vi "차선 인식(선형 피팅).vi"() -> ()   [LabVIEW 2018]
uses:
  <vilib>/Math Plots/3D Math Plots/3D Scatter/3D Scatter XCtrl/3D Scatter.xctl
  <vilib>/Analysis/Matrix/Datatypes/RealMatrix.ctl
  <vilib>/Analysis/Matrix/Numeric/Conversions/Array To Matrix - RA.vi
  <vilib>/Analysis/Matrix/Numeric/Multiply/Multiply - RM,RM.vi
  <vilib>/Analysis/Matrix/Numeric/Conversions/Matrix To Array - RM.vi
  <vilib>/Math Plots/3D Math Plots/3D Scatter/3D Scatter Datatype/Public/Plot Helper (Vector).vi
  <vilib>/Math Plots/3D Math Plots/3D Scatter/3D Scatter Datatype/3D Scatter Datatype.lvclass
  <vilib>/Analysis/Matrix/NI_Matrix.lvlib
  <vilib>/Analysis/NI_AALPro.lvlib
panel:
  out "노이즈 제거 후 오른쪽 차선":cluster{dbl[], dbl[]}(graph)
  out "노이즈 제거 후 전체 차선":cluster{dbl[], dbl[]}(graph)
  out "노이즈 제거 후 왼쪽 차선":cluster{dbl[], dbl[]}(graph)
  out "왼쪽 차선(중점":cluster{dbl[], dbl[]}(graph)
  out "오른쪽 차선(중점)":cluster{dbl[], dbl[]}(graph)
  out "클러스터링 후 (중점)":cluster{dbl[], dbl[]}(graph)
  out "전체 차선":cluster{dbl[], dbl[]}(graph)
  out "왼쪽 차선":cluster{dbl[], dbl[]}(graph)
  out "오른쪽 차선":cluster{dbl[], dbl[]}(graph)
  out "왼쪽 차선(모든 점)":cluster{dbl[], dbl[]}(graph)
  out "오른쪽 차선(모든 점)":cluster{dbl[], dbl[]}(graph)
  out "반사율 꼬깔콘":cluster{dbl[], dbl[]}(graph)
  out "101이상 반사율":u8[](array[numeric])
  out "95~100반사율 배열":cluster{dbl, dbl, dbl, u8}[](array[cluster])
  out "반사율 xy(차선x)":cluster{dbl[], dbl[]}(graph)
  out "60미만 반사율":u8[](array[numeric])
  out "95이상 반사율":u8[](array[numeric])
  out "반사율 xy":cluster{dbl[], dbl[]}(graph)
  out "XZ 2":cluster{dbl[], dbl[]}(graph)
  out "클러스터링 후(모든 점)":cluster{dbl[], dbl[]}(graph)
  out "배열 5":cluster{dbl, dbl, dbl, i32}[](array[cluster])
  out "배열 2":u8[](array[numeric])
  out "XY 그래프":cluster{dbl[], dbl[]}(graph)
  out "azimuth 배열 사이즈":i32
  out "XZ":cluster{dbl[], dbl[]}(graph)
  out "YZ":cluster{dbl[], dbl[]}(graph)
  out "XY":cluster{dbl[], dbl[]}(graph)
  out "3D Scatter":refnum<class "3D Plot Datatype.lvclass">[](xcontrol)
  out "범위내의 X,Y,Z,반사율":cluster{dbl, dbl, dbl, u8}[](array[cluster])
  out "substring":string
  out "Array":string[](array[string])
  out "distance":dbl[](array[numeric])
  out "output array":u8[](array[numeric])
  in  "Boolean":bool
  out "xz":cluster{dbl[], dbl[]}(graph)
  out "yz":cluster{dbl[], dbl[]}(graph)
  out "XY Graph":cluster{dbl[], dbl[]}(graph)
  out "unsigned byte array":u8[][][](array[numeric])
  out "azimuth":dbl[](array[numeric])
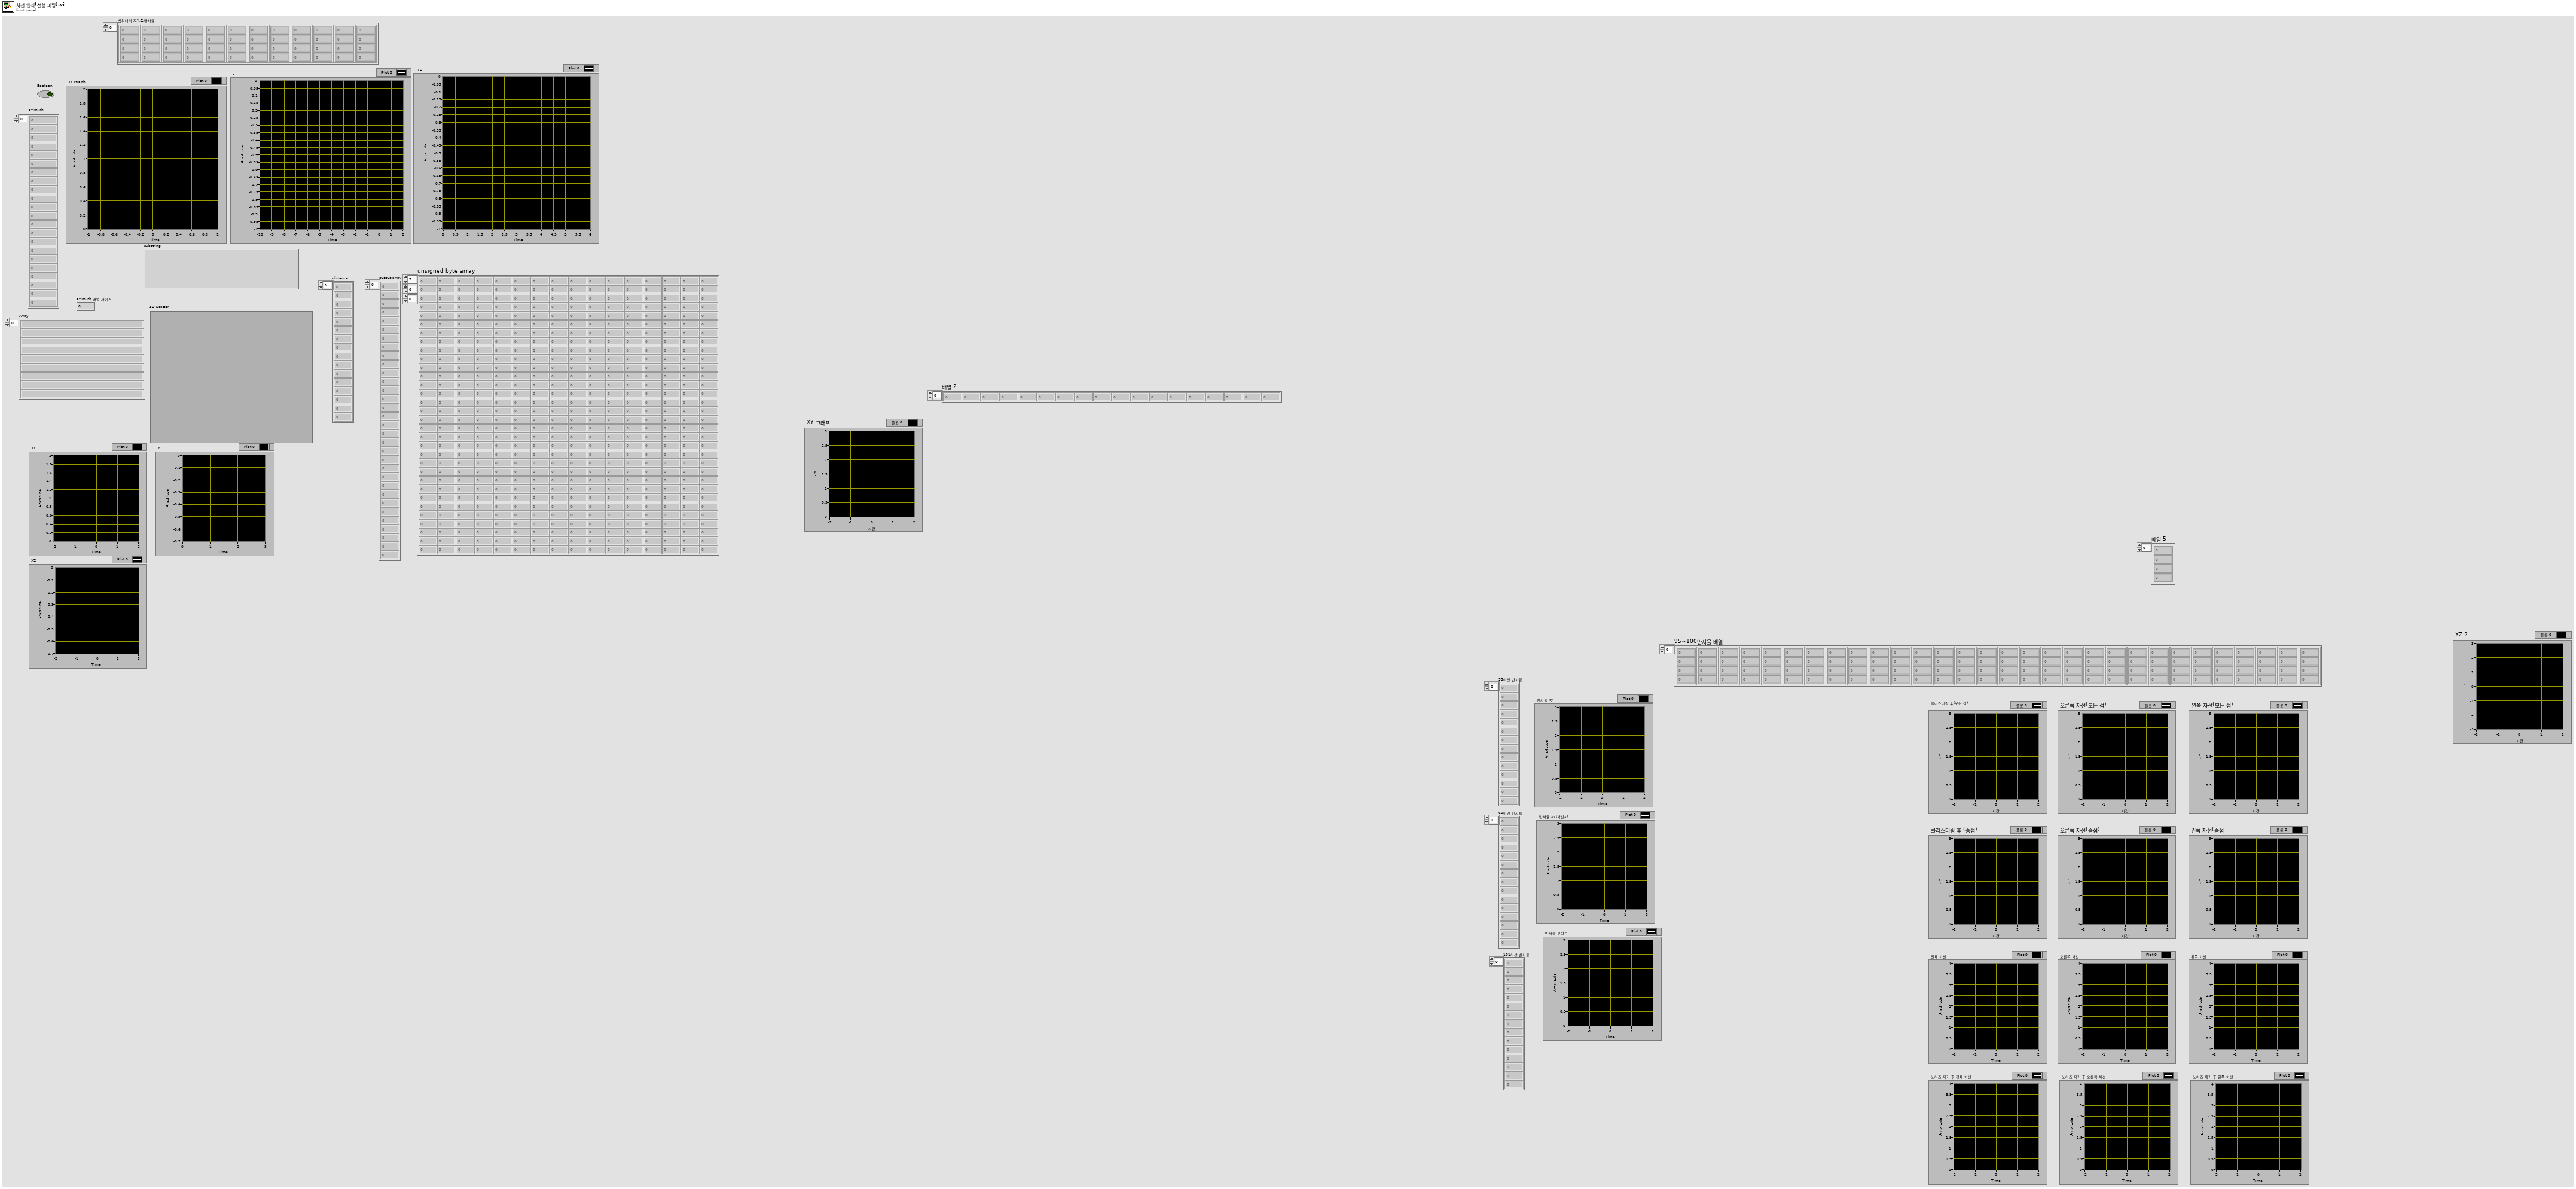
[diagram p1: front panel]
types:
  T1 = typedef "NI_Matrix.lvlib/RealMatrix.ctl" = dbl[][]
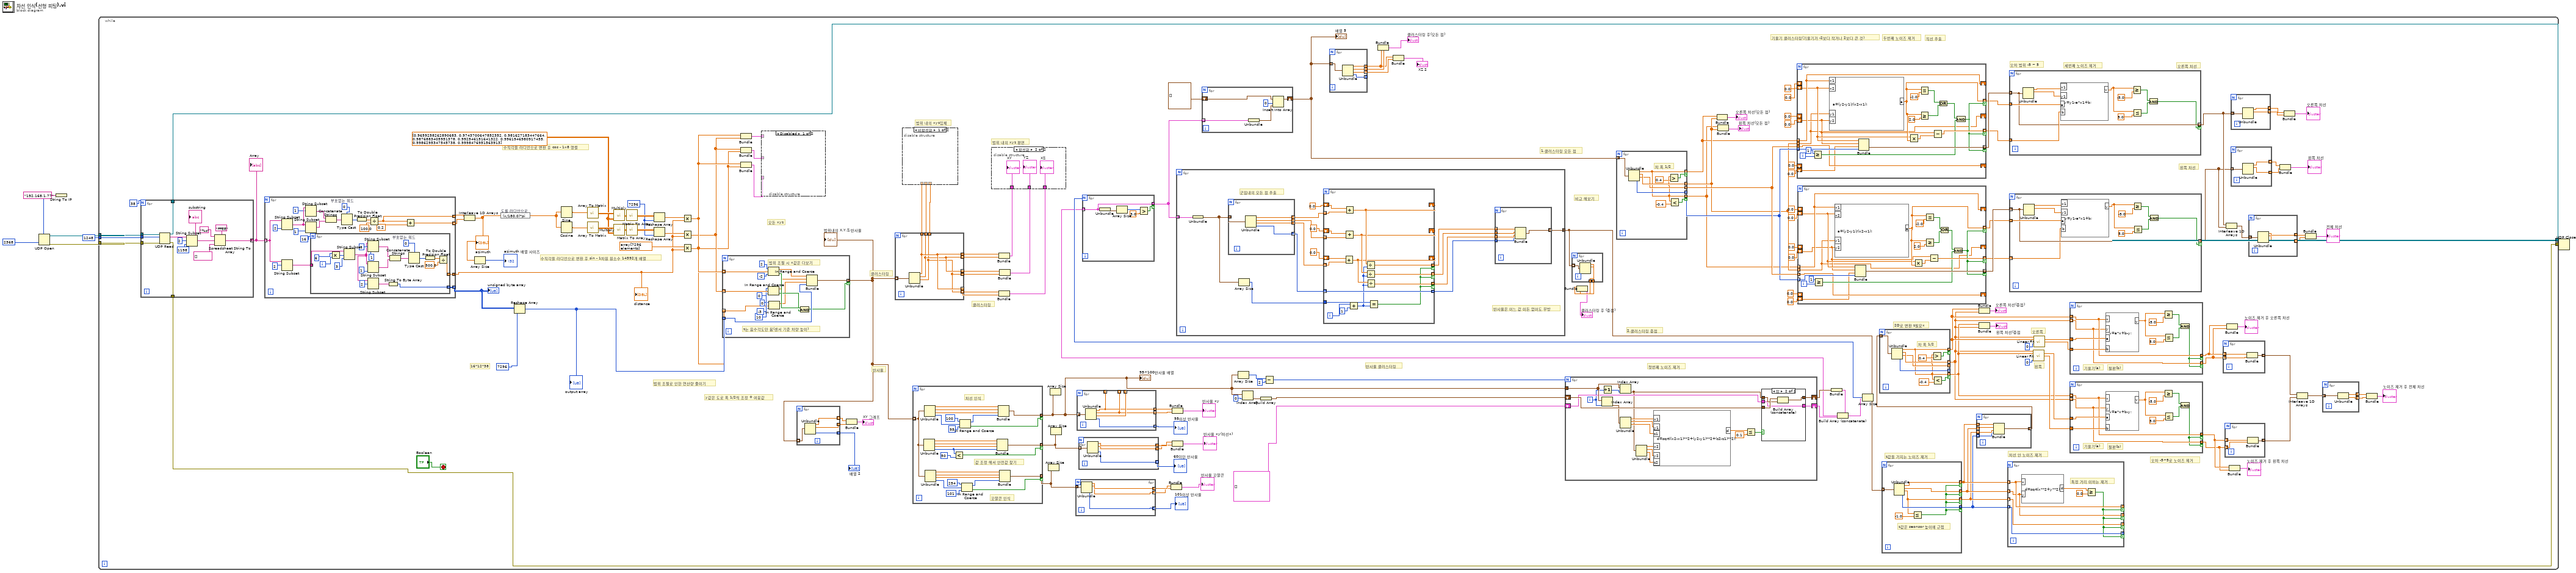
[diagram p0: block diagram]
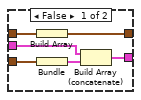
[diagram p2: hidden frame]
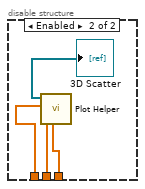
[diagram p4: hidden frame]
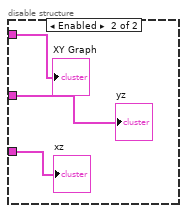
[diagram p5: hidden frame]
diagram:
  n1 = String To IP(1:"192.168.1.77") -> (0:w7:u32)
  n2 = UDP Open(7:w7, 11:2368) -> (port=w5:refnum<k16>, 0:w3:errorcluster)  [unwired: 3 in, 1 out]
  n3 = while {
    tunnel: w5 -> [w164]
    tunnel: 1248 -> [w163]
    tunnel: w3 -> [w162]
    tunnel: [w151] -> w2
    tunnel: [w134] -> w1
    stop <- "Boolean" stop-if-true
    w125 = 7296 ("차원 크기")
    w122 = T1 [[0.9659258262890683, 0.9743700647852352, 0.981627183447664, 0.9876883405951378, 0.992546151641322, 0.9961946980917455, 0.9986295347545738, 0.9998476951563913]] ("전치 행렬")
    # "오차 -5~5로 노이즈 제거"
    # "2D로 변환 z필요x"
    # "왼쪽"
    # "오른쪽"
    # "차선 안 노이즈 제거"
    # "z값을 가지는 노이즈 제거"
    # "2.클러스터링 중점"
    # "1.클러스터링 모든 점"
    # "비교 해보기"
    # "왼쪽 차선"
    # "오른쪽 차선"
    # "오차 범위 -5 ~ 5"
    # "세번째 노이즈 제거"
    # "직선 추출"
    # "기울기 클러스터링(기울기가 -2보다 작거나 2보다 큰 것)"
    # "두번째 노이즈 제거"
    # "첫번째 노이즈 제거"
    # "y값은 도로 폭 1/2씩 조정 + 여윳값"
    # "반사율 클러스터링"
    # "범위 조절로 인한 연산량 줄이기"
    # "반사율"
    # "클러스터링"
    # "수직각을 라디언으로 변환 후 cos - 1x8 행렬"
    # "클러스터링"
    # "범위 내의 xyz 평면"
    # "범위 내의 xyz입체"
    # "모든 xyz"
    # "16*12*38"
    # "수직각을 라디언으로 변환 후 sin - 1차원 원소수 14592개 배열"
    n4 = for {
      N: 38 -> [_]
      tunnel: w164 -> [w518]
      tunnel: w163 -> [w517]
      tunnel: w162 -> [w516]
      tunnel: [w512] -> w151
      tunnel: [w507] -> w161 mode=concatenating
      tunnel: [w506] -> w134
      n5 = UDP Read(connection ID=w518, max size (548)=w517, 8:w516) -> (data out=w515:string, error out=w512:errorcluster, 3:w506:refnum<k16>)  [unwired: 1 in, 2 out]
      n6 = String Subset(string=w515, offset (0)=2, length (rest)=1198) -> (substring=w511:string)
      "substring" <- w511
      n7 = Spreadsheet String To Array(delimiter (Tab)="FFEE", format string="%s", spreadsheet string=w511, array type (2D Dbl)=string[] []) -> (array=w507:string[])
    }
    "Array" <- w161
    n8 = for {
      tunnel: w161 -> [w485] mode=indexing
      tunnel: [w472] -> w159 mode=indexing
      tunnel: [w471] -> w160 mode=indexing
      tunnel: [w468] -> w118 mode=concatenating
      tunnel: [w467] -> w158 mode=indexing
      w466 = u16 0  # 부호없는 워드
      n9 = String Subset(string=w485, offset (0)=2) -> (substring=w469:string)  [unwired: 1 in]
      n10 = String Subset(string=w485, length (rest)=2) -> (substring=w482:string)  [unwired: 1 in]
      n11 = String Subset(string=w482, offset (0)=1) -> (substring=w479:string)  [unwired: 1 in]
      n12 = String Subset(string=w482, length (rest)=1) -> (substring=w478:string)  [unwired: 1 in]
      n13 = for {
        N: 16 -> [_]
        tunnel: w469 -> [w505]
        tunnel: [w492] -> w468 mode=indexing
        tunnel: [w488] -> w467 mode=indexing
        i -> [w504]
        w486 = u16 0  # 부호없는 워드
        n14 = Multiply(x=6, y=w504) -> (x*y=w502:i32)
        n15 = String Subset(string=w505, offset (0)=w502, length (rest)=3) -> (substring=w491:string)
        n16 = String Subset(string=w491, offset (0)=2) -> (substring=w489:string)  [unwired: 1 in]
        n17 = String Subset(string=w491, offset (0)=1, length (rest)=1 ("length (rest)")) -> (substring=w498:string)
        n18 = String Subset(string=w491, length (rest)=1) -> (substring=w497:string)  [unwired: 1 in]
        n19 = String To Byte Array(string=w489) -> (unsigned byte array=w488:u8[])
        n20 = Concatenate Strings(w498, w497) -> (w496:string)
        n21 = Type Cast(type=w486, x=w496) -> (*(type *) &x=w495:u16)
        n22 = To Double Precision Float(number=w495) -> (double precision float=w494:dbl)
        n23 = Divide(x=w494, y=500.0) -> (x/y=w492:dbl)
      }
      n24 = Concatenate Strings(w479, w478) -> (w477:string)
      n25 = Type Cast(type=w466, x=w477) -> (*(type *) &x=w476:u16)
      n26 = To Double Precision Float(number=w476) -> (double precision float=w475:dbl)
      n27 = Divide(x=w475, y=100.0) -> (x/y=w471:dbl)
      n28 = Add(x=w471, y=0.2) -> (x+y=w472:dbl)
    }
    "unsigned byte array" <- w158
    "distance" <- w118
    n29 = Interleave 1D Arrays(w160, w159) -> (w136:dbl[])
    "azimuth" <- w136
    n30 = Array Size(array=w136) -> (size(s)=→"azimuth 배열 사이즈":i32)
    n31 = expression code="(x/180.0)*pi" "도를 라디안으로"(w136) -> (w147:dbl[])
    n32 = Reshape Array(w158, 7296 ("차원 크기")) -> (w156:u8[])
    "output array" <- w156
    n33 = Sine(x=w147) -> (sin(x)=w124:dbl[])
    n34 = Cosine(x=w147) -> (cos(x)=w123:dbl[])
    n35 = call-poly <vilib>:"Array To Matrix.vi"("Real 1D Array"=w124) -> ("Real Matrix (Column Vector)"=w131:T1)
    n36 = call-poly <vilib>:"Array To Matrix.vi"("Real 1D Array"=w123) -> ("Real Matrix (Column Vector)"=w130:T1)
    n37 = call-poly <vilib>:"Multiply.vi"("Real Matrix B"=w122, "Real Matrix A"=w131) -> ("A * B"=w129:T1)
    n38 = call-poly <vilib>:"Multiply.vi"("Real Matrix B"=w122, "Real Matrix A"=w130) -> ("A * B"=w128:T1)
    n39 = call-poly <vilib>:"Matrix To Array.vi"("Real Matrix"=w129) -> ("Real 2D Array"=w127:dbl[][])
    n40 = call-poly <vilib>:"Matrix To Array.vi"("Real Matrix"=w128) -> ("Real 2D Array"=w126:dbl[][])
    n41 = Reshape Array(w127, w125) -> (w121:dbl[])
    n42 = Reshape Array(w126, w125) -> (w120:dbl[])
    n43 = Multiply ("Multiply.vi")(x=w121, y=w118) -> (x*y=w150:dbl[])
    n44 = Multiply ("Multiply.vi")(x=w120, y=w118) -> (x*y=w149:dbl[])
    n45 = Multiply ("Multiply.vi")(x=dbl[] array[7296 elements] ("배열 2"), y=w118) -> (x*y=w148:dbl[])
    n46 = for {
      tunnel: w150 -> [w465] mode=indexing
      tunnel: w149 -> [w464] mode=indexing
      tunnel: w148 -> [w453] mode=indexing
      tunnel: w156 -> [w456] mode=indexing
      tunnel: [w455] -> w81 mode=indexing if=w454
      # "범위 조절 시 x값은 다보기"
      # "z는 음수각도만 봄(센서 기준 차량 높이)"
      n47 = In Range and Coerce(upper limit=2, x=w465, lower limit=-2) -> (coerced(x)=w458:dbl, In Range?=w460:bool)
      n48 = In Range and Coerce(upper limit=10, x=w464, lower limit=0) -> (coerced(x)=w457:dbl, In Range?=w459:bool)
      n49 = In Range and Coerce(upper limit=0, x=w453, lower limit=-3) -> (coerced(x)=w451:dbl)  [unwired: 1 out]
      n50 = Compound Arithmetic op=AND(w460, w459) -> (w454:bool)
      n51 = Bundle(w458, w457, w451, w456) -> (w455:cluster{dbl, dbl, dbl, u8})  [unwired: 1 in]
    }
    "범위내의 X,Y,Z,반사율" <- w81
    n52 = Bundle(w150, w149) -> (w155:cluster{dbl[], dbl[]})  [unwired: 1 in]
    n53 = Bundle(w149, w148) -> (w154:cluster{dbl[], dbl[]})  [unwired: 1 in]
    n54 = Bundle(w150, w148) -> (w153:cluster{dbl[], dbl[]})  [unwired: 1 in]
    n55 = disable-structure shown="Disabled" {
      disable-tunnel: w155 -> [_ w448]
      disable-tunnel: w154 -> [_ w447]
      disable-tunnel: w153 -> [_ w446]
      frame Disabled {
      }
      frame Enabled {
        "XY Graph" <- w448
        "yz" <- w447
        "xz" <- w446
      }
    }
    n56 = for {
      tunnel: w81 -> [w434] mode=indexing
      tunnel: [w433] -> w117 mode=indexing
      tunnel: [w432] -> w115 mode=indexing
      tunnel: [w431] -> w114 mode=indexing
      n57 = Unbundle(w434) -> (w433:dbl, w432:dbl, w431:u8)  [unwired: 1 out]
    }
    "배열 2" <- w114
    n58 = Bundle(w117, w115) -> (→"XY 그래프":cluster{dbl[], dbl[]})  [unwired: 1 in]
    n59 = for {
      tunnel: w81 -> [w445] mode=indexing
      tunnel: [w444] -> w133 mode=indexing
      tunnel: [w443] -> w132 mode=indexing
      tunnel: [w442] -> w146 mode=indexing
      tunnel: [w443] -> w145 mode=indexing
      tunnel: [w444] -> w144 mode=indexing
      tunnel: [w442] -> w143 mode=indexing
      tunnel: [w444] -> w142 mode=indexing
      tunnel: [w443] -> w141 mode=indexing
      tunnel: [w442] -> w140 mode=indexing
      n60 = Unbundle(w445) -> (w444:dbl, w443:dbl, w442:dbl)  [unwired: 1 out]
    }
    n61 = disable-structure shown="비활성화" {
      disable-tunnel: w142 -> [_ w440]
      disable-tunnel: w141 -> [_ w439]
      disable-tunnel: w140 -> [_ w438]
      frame Disabled {
      }
      frame Enabled {
        n62 = call-poly <vilib>:"Plot Helper.vi"("z vector"=w438, "y vector"=w439, "x vector"=w440) -> ("3D Plot lvclass Array out"=→"3D Scatter":refnum<class "3D Plot Datatype.lvclass">[])  [unwired: 3 in, 5 out]
      }
    }
    n63 = for {
      tunnel: w81 -> [w376] mode=indexing
      tunnel: [w384] -> w80 mode=indexing if=w371
      tunnel: [w380] -> w91 mode=indexing if=w377
      tunnel: [w372] -> w86 mode=indexing if=w362
      # "꼬깔콘 인식"
      # "차선 인식"
      # "값 조정 해서 안전값 찾기"
      n64 = Unbundle(w376) -> (w383:dbl, w382:dbl, w381:dbl, w379:u8)
      n65 = Unbundle(w376) -> (w387:dbl, w386:dbl, w385:dbl, w370:u8)
      n66 = Unbundle(w376) -> (w375:dbl, w374:dbl, w373:dbl, w366:u8)
      n67 = Less?(x=w379, y=50) -> (x < y?=w377:bool)
      n68 = In Range and Coerce(upper limit=100, x=w370, lower limit=95) -> (coerced(x)=w369:i32, In Range?=w371:bool)
      n69 = In Range and Coerce(upper limit=254, x=w366, lower limit=101) -> (coerced(x)=w363:i32, In Range?=w362:bool)
      n70 = Bundle(w383, w382, w381, w379) -> (w380:cluster{dbl, dbl, dbl, u8})  [unwired: 1 in]
      n71 = Bundle(w387, w386, w385, w369) -> (w384:cluster{dbl, dbl, dbl, i32})  [unwired: 1 in]
      n72 = Bundle(w375, w374, w373, w363) -> (w372:cluster{dbl, dbl, dbl, i32})  [unwired: 1 in]
    }
    "95~100반사율 배열" <- w80
    n73 = Bundle(w133, w132) -> (w139:cluster{dbl[], dbl[]})  [unwired: 1 in]
    n74 = Bundle(w144, w143) -> (w137:cluster{dbl[], dbl[]})  [unwired: 1 in]
    n75 = Bundle(w145, w146) -> (w138:cluster{dbl[], dbl[]})  [unwired: 1 in]
    n76 = disable-structure shown="활성화" {
      disable-tunnel: w139 -> [_ w435]
      disable-tunnel: w138 -> [_ w437]
      disable-tunnel: w137 -> [_ w436]
      frame Disabled {
      }
      frame Enabled {
        "XY" <- w435
        "YZ" <- w437
        "XZ" <- w436
      }
    }
    n77 = Array Size(array=w86) -> ()  [unwired: 1 out]
    n78 = Array Size(array=w80) -> ()  [unwired: 1 out]
    n79 = Array Size(array=w91) -> ()  [unwired: 1 out]
    n80 = for {
      tunnel: w86 -> [w352] mode=indexing
      tunnel: [w351] -> w85 mode=indexing
      tunnel: [w350] -> w84 mode=indexing
      tunnel: [w349] -> w83 mode=indexing
      n81 = Unbundle(w352) -> (w351:dbl, w350:dbl, w349:i32)  [unwired: 1 out]
    }
    "101이상 반사율" <- w83
    n82 = for {
      tunnel: [w357] -> w95 mode=indexing
      tunnel: [w358] -> w94 mode=indexing
      tunnel: [w361] -> w92 mode=indexing
      tunnel: w80 -> [w360] mode=indexing
      tunnel: [w359] -> _ mode=indexing
      tunnel: [w358] -> _ mode=indexing
      tunnel: [w357] -> _ mode=indexing
      n83 = Unbundle(w360) -> (w357:dbl, w358:dbl, w359:dbl, w361:i32)
    }
    "95이상 반사율" <- w92
    n84 = for {
      tunnel: w91 -> [w356] mode=indexing
      tunnel: [w355] -> w90 mode=indexing
      tunnel: [w354] -> w89 mode=indexing
      tunnel: [w353] -> w88 mode=indexing
      n85 = Unbundle(w356) -> (w354:dbl, w353:dbl, w355:u8)  [unwired: 1 out]
    }
    "60미만 반사율" <- w90
    n86 = Bundle(w85, w84) -> (→"반사율 꼬깔콘":cluster{dbl[], dbl[]})  [unwired: 1 in]
    n87 = Bundle(w95, w94) -> (→"반사율 xy":cluster{dbl[], dbl[]})  [unwired: 1 in]
    n88 = Bundle(w89, w88) -> (→"반사율 xy(차선x)":cluster{dbl[], dbl[]})  [unwired: 1 in]
    n89 = Array Size(array=w80) -> (size(s)=w113:i32)
    n90 = Index Array(array=w80, index=0 ("인덱스")) -> (element=w110:cluster{dbl, dbl, dbl, i32})
    n91 = Build Array(w110) -> (w111:cluster{dbl, dbl, dbl, i32}[])
    n92 = Subtract(x=w113, y=2) -> (x-y=w108:i32)
    n93 = for {
      N: w108 -> [_]
      tunnel: w80 -> [w419]
      shift-right: [w403] -> w99
      shift-left: w111 -> [w409]
      shift-right: [w407] -> w98
      shift-left: cluster{cluster{dbl, dbl, dbl, u8}[]}[] [] -> [w408]
      i -> [w404]
      n94 = Index Array(array=w419, index=w404) -> (element=w406:cluster{dbl, dbl, dbl, i32})
      n95 = Increment(x=w404) -> (x+1=w420:i32)
      n96 = Index Array(array=w419, index=w420) -> (element=w405:cluster{dbl, dbl, dbl, i32})
      n97 = Unbundle(w406) -> (w418:dbl, w417:dbl, w416:dbl)  [unwired: 1 out]
      n98 = Unbundle(w405) -> (w415:dbl, w414:dbl, w413:dbl)  [unwired: 1 out]
      n99 = formula code="d=sqrt((x2-x1)**2+(y2-y1)**2+(z2-z1)**2);"("x1"=w418, "y1"=w417, "z1"=w416, "x2"=w415, "y2"=w414, "z2"=w413) -> ("d"=w412:dbl)
      n100 = Less Or Equal?(x=w412, y=0.1) -> (x <= y?=w410:bool)
      n101 = case shown="참" w410 {
        tunnel: w409 -> [w426 w430]
        tunnel: w405 -> [w422 w429]
        tunnel: w408 -> [w425 w428]
        tunnel: [w423 w428] -> w407
        tunnel: [w421 w427] -> w403
        frame False {
          n102 = Build Array(w422) -> (w421:cluster{dbl, dbl, dbl, i32}[])
          n103 = Bundle(w426) -> (w424:cluster{cluster{dbl, dbl, dbl, i32}[]})  [unwired: 1 in]
          n104 = Build Array (concatenate)(w425, w424) -> (w423:cluster{cluster{dbl, dbl, dbl, i32}[]}[])
        }
        frame True {
          n105 = Build Array (concatenate)(w430, w429) -> (w427:cluster{dbl, dbl, dbl, i32}[])
        }
      }
    }
    n106 = Bundle(w99) -> (w100:cluster{cluster{dbl, dbl, dbl, i32}[]})  [unwired: 1 in]
    n107 = Build Array (concatenate)(w100, w98) -> (w96:cluster{cluster{dbl, dbl, dbl, i32}[]}[])
    n108 = Array Size(array=w96) -> (size(s)=w97:i32)
    n109 = for {
      N: w97 -> [_]
      tunnel: w96 -> [w398] mode=indexing
      tunnel: [w398] -> w43 mode=indexing if=w400
      n110 = Unbundle(w398) -> (w399:cluster{dbl, dbl, dbl, i32}[])
      n111 = Array Size(array=w399) -> (size(s)=w401:i32)
      n112 = Greater?(x=w401, y=3.0) -> (0:w400:bool)
    }
    n113 = for {
      tunnel: w43 -> [w228] mode=indexing
      tunnel: [w231] -> w26 mode=concatenating
      # "반사율은 어느 값 이든 없어도 무방"
      # "군집내의 모든 점 추출"
      n114 = Unbundle(w228) -> (w227:cluster{dbl, dbl, dbl, i32}[])
      n115 = for {
        tunnel: [w268] -> w240 mode=indexing
        tunnel: [w267] -> w239 mode=indexing
        tunnel: [w266] -> w238 mode=indexing
        tunnel: [w265] -> w234 mode=indexing
        tunnel: w227 -> [w264] mode=indexing
        n116 = Unbundle(w264) -> (w268:dbl, w267:dbl, w266:dbl, w265:i32)
      }
      n117 = Array Size(array=w227) -> (size(s)=w226:i32)
      n118 = for {
        shift-right: [w256] -> _
        shift-left: 0.0 -> [w263]
        shift-right: [w255] -> _
        shift-left: 0.0 -> [w261]
        shift-right: [w254] -> _
        shift-left: 0.0 -> [w259]
        tunnel: w240 -> [w262] mode=indexing
        tunnel: w239 -> [w260] mode=indexing
        tunnel: w238 -> [w258] mode=indexing
        tunnel: w234 -> [w257] mode=indexing
        tunnel: [w257] -> w232 mode=indexing
        tunnel: [w253] -> w230 mode=indexing if=w248
        tunnel: [w252] -> w229 mode=indexing if=w248
        tunnel: [w251] -> w233 mode=indexing if=w248
        tunnel: w226 -> [w247]
        i -> [w250]
        n119 = Add(x=w259, y=w258) -> (x+y=w254:dbl)
        n120 = Add(x=w261, y=w260) -> (x+y=w255:dbl)
        n121 = Add(x=w263, y=w262) -> (x+y=w256:dbl)
        n122 = Add(x=w250, y=1) -> (x+y=w246:i32)
        n123 = Divide(x=w256, y=w246) -> (x/y=w253:dbl)
        n124 = Divide(x=w255, y=w246) -> (x/y=w252:dbl)
        n125 = Divide(x=w254, y=w246) -> (x/y=w251:dbl)
        n126 = Equal?(x=w247, y=w246) -> (x = y?=w248:bool)
      }
      n127 = for {
        tunnel: w230 -> [w245] mode=indexing
        tunnel: w229 -> [w244] mode=indexing
        tunnel: w233 -> [w243] mode=indexing
        tunnel: w232 -> [w242] mode=indexing
        tunnel: [w241] -> w231 mode=indexing
        n128 = Bundle(w245, w244, w243, w242) -> (w241:cluster{dbl, dbl, dbl, i32})  [unwired: 1 in]
      }
    }
    n129 = for {
      shift-right: [w397] -> w40
      shift-left: cluster{dbl, dbl, dbl, i32}[] [] -> [w396]
      tunnel: w43 -> [w393] mode=indexing
      n130 = Unbundle(w393) -> (w395:cluster{dbl, dbl, dbl, i32}[])
      n131 = Insert Into Array(array=w396, index=0 ("인덱스"), new element=w395) -> (w397:cluster{dbl, dbl, dbl, i32}[])
    }
    "배열 5" <- w40
    n132 = for {
      tunnel: w40 -> [w392] mode=indexing
      tunnel: [w391] -> w102 mode=indexing
      tunnel: [w390] -> w105 mode=indexing
      tunnel: [w389] -> w103 mode=indexing
      tunnel: [w388] -> _ mode=indexing
      n133 = Unbundle(w392) -> (w391:dbl, w390:dbl, w389:dbl, w388:i32)
    }
    n134 = Bundle(w102, w105) -> (→"클러스터링 후(모든 점)":cluster{dbl[], dbl[]})  [unwired: 1 in]
    n135 = Bundle(w102, w103) -> (→"XZ 2":cluster{dbl[], dbl[]})  [unwired: 1 in]
    n136 = for {
      tunnel: w26 -> [w216] mode=indexing
      tunnel: [w215] -> w46 mode=indexing
      tunnel: [w214] -> w45 mode=indexing
      n137 = Unbundle(w216) -> (w215:dbl, w214:dbl)  [unwired: 2 out]
    }
    n138 = Bundle(w46, w45) -> (→"클러스터링 후 (중점)":cluster{dbl[], dbl[]})  [unwired: 1 in]
    n139 = for {
      tunnel: w40 -> [w348] mode=indexing
      tunnel: [w341] -> w68 mode=indexing if=w347
      tunnel: [w346] -> w69 mode=indexing
      tunnel: [w345] -> w77 mode=indexing
      tunnel: [w344] -> w76 mode=indexing
      tunnel: [w341] -> w55 mode=indexing if=w343
      # "차 폭 1/2"
      n140 = Unbundle(w348) -> (w341:dbl, w346:dbl, w345:dbl, w344:i32)
      n141 = Greater?(x=w341, y=0.4) -> (0:w347:bool)
      n142 = Less?(x=w341, y=-0.4) -> (x < y?=w343:bool)
    }
    n143 = Bundle(w68, w69) -> (→"오른쪽 차선(모든 점)":cluster{dbl[], dbl[]})  [unwired: 1 in]
    n144 = Bundle(w55, w69) -> (→"왼쪽 차선(모든 점)":cluster{dbl[], dbl[]})  [unwired: 1 in]
    n145 = for {
      shift-right: [w330] -> _
      shift-left: 0.0 -> [_]
      shift-right: [w322] -> _
      shift-left: 0.0 -> [_]
      shift-left: 0.0 -> [w324]
      shift-left: 0.0 -> [w323]
      tunnel: w77 -> [w321] mode=indexing
      tunnel: w76 -> [w337] mode=indexing
      tunnel: [w336] -> w75 mode=indexing if=w325
      tunnel: [w333] -> w74 mode=indexing if=w325
      tunnel: [w331] -> w73 mode=indexing if=w325
      tunnel: w69 -> [w322] mode=indexing
      tunnel: w68 -> [w330] mode=indexing
      shift-right: [w321] -> _
      shift-left: 0.0 -> [_]
      shift-left: 0.0 -> [w320]
      i -> [w328]
      n146 = Greater Or Equal?(x=1, y=w328) -> (x >= y?=w327:bool)
      n147 = formula code="a=(y2-y1)/(x2-x1);"("x1"=w330, "x2"=w324, "y1"=w322, "y2"=w323) -> ("a"=w333:dbl)
      n148 = Bundle(w324, w323, w320, w337) -> (w336:cluster{dbl, dbl, dbl, i32})  [unwired: 1 in]
      n149 = Multiply(x=w324, y=w333) -> (x*y=w332:dbl)
      n150 = Less Or Equal?(x=w333, y=-2.0) -> (x <= y?=w335:bool)
      n151 = Greater Or Equal?(x=w333, y=2.0) -> (x >= y?=w334:bool)
      n152 = Subtract(x=w323, y=w332) -> (x-y=w331:dbl)
      n153 = Or(x=w335, y=w334) -> (x .or. y?=w326:bool)
      n154 = And(x=w326, y=w327) -> (x .and. y?=w325:bool)
    }
    n155 = for {
      shift-right: [w310] -> _
      shift-left: 0.0 -> [_]
      shift-right: [w302] -> _
      shift-left: 0.0 -> [_]
      shift-left: 0.0 -> [w303]
      shift-left: 0.0 -> [w304]
      tunnel: w77 -> [w301] mode=indexing
      tunnel: w76 -> [w317] mode=indexing
      tunnel: [w316] -> w72 mode=indexing if=w305
      tunnel: [w313] -> w71 mode=indexing if=w305
      tunnel: [w311] -> w70 mode=indexing if=w305
      tunnel: w55 -> [w310] mode=indexing
      tunnel: w69 -> [w302] mode=indexing
      shift-right: [w301] -> _
      shift-left: 0.0 -> [_]
      shift-left: 0.0 -> [w300]
      i -> [w308]
      n156 = Greater Or Equal?(x=1, y=w308) -> (x >= y?=w306:bool)
      n157 = formula code="a=(y2-y1)/(x2-x1);"("x1"=w310, "x2"=w304, "y1"=w302, "y2"=w303) -> ("a"=w313:dbl)
      n158 = Bundle(w304, w303, w300, w317) -> (w316:cluster{dbl, dbl, dbl, i32})  [unwired: 1 in]
      n159 = Multiply(x=w304, y=w313) -> (x*y=w312:dbl)
      n160 = Less Or Equal?(x=w313, y=-2.0) -> (x <= y?=w315:bool)
      n161 = Greater Or Equal?(x=w313, y=2.0) -> (x >= y?=w314:bool)
      n162 = Subtract(x=w303, y=w312) -> (x-y=w311:dbl)
      n163 = Or(x=w315, y=w314) -> (x .or. y?=w307:bool)
      n164 = And(x=w307, y=w306) -> (x .and. y?=w305:bool)
    }
    n165 = for {
      tunnel: w26 -> [w213] mode=indexing
      tunnel: [w212] -> w30 mode=indexing if=w207
      tunnel: [w210] -> w29 mode=indexing if=w207
      tunnel: [w208] -> w28 mode=indexing if=w207
      tunnel: [w209] -> w27 mode=indexing if=w207
      # "z값은 seonsor 높이에 근접"
      n166 = Unbundle(w213) -> (w212:dbl, w210:dbl, w208:dbl, w209:i32)
      n167 = Less Or Equal?(x=w208, y=-1.0) -> (x <= y?=w207:bool)
    }
    n168 = for {
      tunnel: w30 -> [w189] mode=indexing
      tunnel: w29 -> [w188] mode=indexing
      tunnel: w28 -> [w187] mode=indexing
      tunnel: w27 -> [w186] mode=indexing
      tunnel: [w185] -> w25 mode=indexing
      n169 = Bundle(w189, w188, w187, w186) -> (w185:cluster{dbl, dbl, dbl, i32})  [unwired: 1 in]
    }
    n170 = for {
      tunnel: w25 -> [w217] mode=indexing
      tunnel: [w219] -> w31 mode=indexing if=w225
      tunnel: [w224] -> w21 mode=indexing
      tunnel: [w223] -> _ mode=indexing
      tunnel: [w222] -> _ mode=indexing
      tunnel: [w219] -> w22 mode=indexing if=w221
      # "차 폭 1/2"
      n171 = Unbundle(w217) -> (w219:dbl, w224:dbl, w223:dbl, w222:i32)
      n172 = Greater?(x=w219, y=0.4) -> (0:w225:bool)
      n173 = Less?(x=w219, y=-0.4) -> (x < y?=w221:bool)
    }
    n174 = Bundle(w31, w21) -> (→"오른쪽 차선(중점)":cluster{dbl[], dbl[]})  [unwired: 1 in]
    n175 = Bundle(w22, w21) -> (→"왼쪽 차선(중점":cluster{dbl[], dbl[]})  [unwired: 1 in]
    n176 = for {
      tunnel: w30 -> [w206] mode=indexing
      tunnel: w29 -> [w205] mode=indexing
      tunnel: w28 -> [w204] mode=indexing
      tunnel: w27 -> [w203] mode=indexing
      tunnel: [w206] -> _ mode=indexing if=w202
      tunnel: [w205] -> _ mode=indexing if=w202
      tunnel: [w204] -> _ mode=indexing if=w202
      tunnel: [w203] -> _ mode=indexing if=w202
      # "특정 거리 이하는 제거"
      n177 = formula code="d=sqrt(x**2+y**2);"("x"=w206, "y"=w205) -> ("d"=w201:dbl)
      n178 = Greater Or Equal?(x=w201, y=0.0) -> (x >= y?=w202:bool)
    }
    n179 = for {
      tunnel: w75 -> [w290] mode=indexing
      tunnel: w74 -> [w297] mode=indexing
      tunnel: w73 -> [w296] mode=indexing
      tunnel: [w290] -> w61 mode=indexing if=w289
      n180 = Unbundle(w290) -> (w299:dbl, w298:dbl)  [unwired: 2 out]
      n181 = formula code="v=y1-a*x1+b;"("x1"=w299, "y1"=w298, "a"=w297, "b"=w296) -> ("v"=w294:dbl)
      n182 = Greater Or Equal?(x=w294, y=-5.0) -> (x >= y?=w292:bool)
      n183 = Less Or Equal?(x=w294, y=5.0) -> (x <= y?=w291:bool)
      n184 = And(x=w292, y=w291) -> (x .and. y?=w289:bool)
    }
    n185 = for {
      tunnel: w72 -> [w280] mode=indexing
      tunnel: w71 -> [w286] mode=indexing
      tunnel: [w280] -> w60 mode=indexing if=w279
      tunnel: w70 -> [w278] mode=indexing
      n186 = Unbundle(w280) -> (w288:dbl, w287:dbl)  [unwired: 2 out]
      n187 = formula code="v=y1-a*x1+b;"("x1"=w288, "y1"=w287, "a"=w286, "b"=w278) -> ("v"=w284:dbl)
      n188 = Greater Or Equal?(x=w284, y=-5.0) -> (x >= y?=w282:bool)
      n189 = Less Or Equal?(x=w284, y=5.0) -> (x <= y?=w281:bool)
      n190 = And(x=w282, y=w281) -> (x .and. y?=w279:bool)
    }
    n191 = call <vilib>:"Linear Fit.vi"("Y"=w21, "X"=w22, "method"=0) -> ("slope"=w24:dbl, "intercept"=w23:dbl)  [unwired: 8 in, 3 out]
    n192 = call <vilib>:"Linear Fit.vi"("Y"=w21, "X"=w31, "tolerance"=0) -> ("slope"=w33:dbl, "intercept"=w32:dbl)  [unwired: 8 in, 3 out]
    n193 = for {
      tunnel: w33 -> [w199]
      tunnel: w32 -> [w198]
      tunnel: w31 -> [w192] mode=indexing
      tunnel: w21 -> [w191] mode=indexing
      tunnel: [w192] -> w17 mode=indexing if=w190
      tunnel: [w191] -> w16 mode=indexing if=w190
      # "절편(b)"
      # "기울기(a)"
      n194 = formula code="v=a*x+b-y;"("x"=w192, "y"=w191, "a"=w199, "b"=w198) -> ("v"=w193:dbl)
      n195 = Greater Or Equal?(x=w193, y=-5.0) -> (x >= y?=w195:bool)
      n196 = Less Or Equal?(x=w193, y=5.0) -> (x <= y?=w194:bool)
      n197 = And(x=w195, y=w194) -> (x .and. y?=w190:bool)
    }
    n198 = for {
      tunnel: w24 -> [w184]
      tunnel: w23 -> [w183]
      tunnel: w22 -> [w177] mode=indexing
      tunnel: w21 -> [w176] mode=indexing
      tunnel: [w177] -> w14 mode=indexing if=w175
      tunnel: [w176] -> w13 mode=indexing if=w175
      # "절편(b)"
      # "기울기(a)"
      n199 = formula code="v=a*x+b-y;"("x"=w177, "y"=w176, "a"=w184, "b"=w183) -> ("v"=w178:dbl)
      n200 = Greater Or Equal?(x=w178, y=-5.0) -> (x >= y?=w180:bool)
      n201 = Less Or Equal?(x=w178, y=5.0) -> (x <= y?=w179:bool)
      n202 = And(x=w180, y=w179) -> (x .and. y?=w175:bool)
    }
    n203 = for {
      tunnel: w17 -> [w174] mode=indexing
      tunnel: w16 -> [w173] mode=indexing
      tunnel: [w172] -> w19 mode=indexing
      n204 = Bundle(w174, w173) -> (w172:cluster{dbl, dbl})  [unwired: 1 in]
    }
    n205 = for {
      tunnel: w14 -> [w171] mode=indexing
      tunnel: w13 -> [w170] mode=indexing
      tunnel: [w169] -> w18 mode=indexing
      n206 = Bundle(w171, w170) -> (w169:cluster{dbl, dbl})  [unwired: 1 in]
    }
    n207 = Interleave 1D Arrays(w61, w60) -> (w59:cluster{dbl, dbl, dbl, i32}[])
    n208 = Bundle(w17, w16) -> (→"노이즈 제거 후 오른쪽 차선":cluster{dbl[], dbl[]})  [unwired: 1 in]
    n209 = Bundle(w14, w13) -> (→"노이즈 제거 후 왼쪽 차선":cluster{dbl[], dbl[]})  [unwired: 1 in]
    n210 = for {
      tunnel: w60 -> [w274] mode=indexing
      tunnel: [w273] -> w64 mode=indexing
      tunnel: [w272] -> w63 mode=indexing
      n211 = Unbundle(w274) -> (w273:dbl, w272:dbl)  [unwired: 2 out]
    }
    n212 = for {
      tunnel: w61 -> [w277] mode=indexing
      tunnel: [w276] -> w67 mode=indexing
      tunnel: [w275] -> w66 mode=indexing
      n213 = Unbundle(w277) -> (w276:dbl, w275:dbl)  [unwired: 2 out]
    }
    n214 = for {
      tunnel: w59 -> [w271] mode=indexing
      tunnel: [w270] -> w58 mode=indexing
      tunnel: [w269] -> w57 mode=indexing
      n215 = Unbundle(w271) -> (w270:dbl, w269:dbl)  [unwired: 2 out]
    }
    n216 = Bundle(w64, w63) -> (→"왼쪽 차선":cluster{dbl[], dbl[]})  [unwired: 1 in]
    n217 = Bundle(w67, w66) -> (→"오른쪽 차선":cluster{dbl[], dbl[]})  [unwired: 1 in]
    n218 = Interleave 1D Arrays(w19, w18) -> (w20:cluster{dbl, dbl}[])
    n219 = Bundle(w58, w57) -> (→"전체 차선":cluster{dbl[], dbl[]})  [unwired: 1 in]
    n220 = for {
      tunnel: w20 -> [w168] mode=indexing
      tunnel: [w167] -> w11 mode=indexing
      tunnel: [w166] -> w10 mode=indexing
      n221 = Unbundle(w168) -> (w167:dbl, w166:dbl)
    }
    n222 = Bundle(w11, w10) -> (→"노이즈 제거 후 전체 차선":cluster{dbl[], dbl[]})  [unwired: 1 in]
  }
  n223 = UDP Close(connection ID=w1, 8:w2) -> ()  [unwired: 2 out]
